vi "GEvt-Filter Global Log - v1.0.vi"(7 "Rules-v1":T1, 11 "Cross CSM Data (in)":T4) -> (0 "Matched? (dup)":bool, 3 "Cross CSM Data":T4)   [LabVIEW 2020, in "Communicable State Machine.lvlib"]
uses:
  Communicable State Machine.lvlib
  _CSM_GlobalLog_MSG.ctl
  _CSM_Response Source Message.ctl
  _CSM_GlobalLog_MSG_TYPE.ctl
  _CSM_GlobalLog Filter Rules - v1.0.ctl
  _CSM_GlobalLog_STATE_TYPE.ctl
  Set Global CSM Filter.vi
  Set Global LogType Filter.vi
  Set Global State Filter.vi
  Set CSM LogType Filter.vi
  Set CSM State Filter.vi
  Set Global StateType Filter.vi
  Set CSM StateType Filter.vi
  Group Check - CSM.vi
  Group Check - LogType.vi
  Group Check - State.vi
  CSM Check - LogType.vi
  CSM Check - State.vi
  CSM Check - StateType.vi
  Group Check - StateType.vi
  LogFilter.lvclass
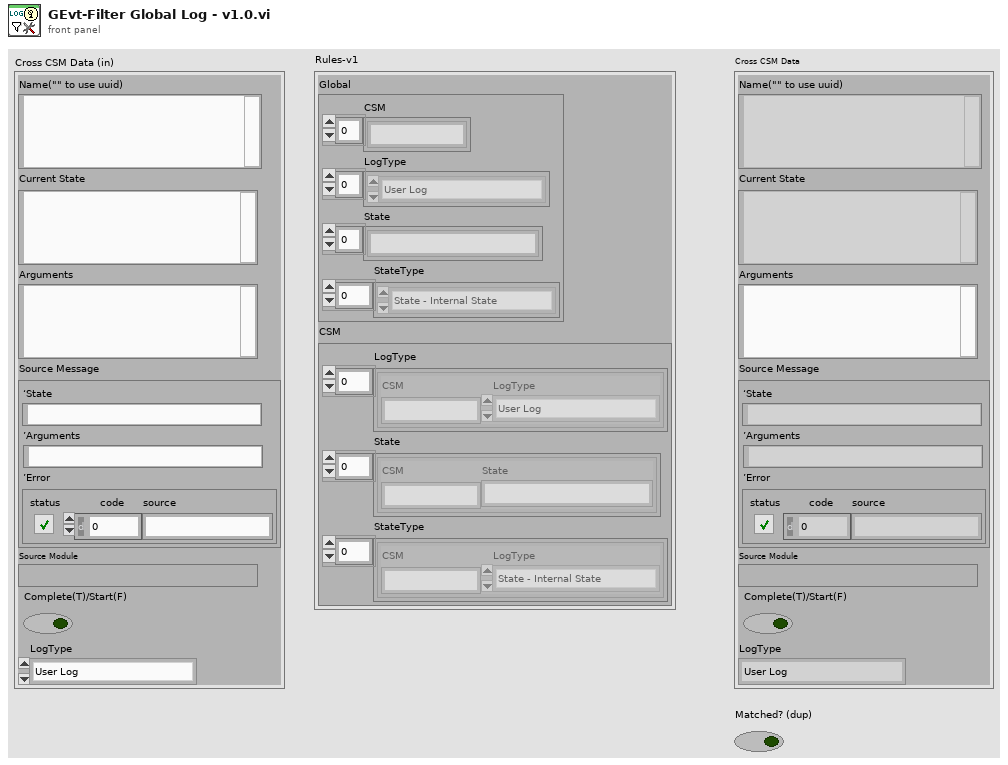
[diagram p1: front panel]
types:
  T1 = typedef "Communicable State Machine.lvlib/_CSM_GlobalLog Filter Rules - v1.0.ctl" = cluster{"Global":cluster{"CSM":string[], "LogType":T2[], "State":string[], "StateType":T3[]}, "CSM":cluster{"LogType":cluster{"CSM":string, "LogType":T2}[], "State":cluster{"CSM":string, "State":string}[], "StateType":cluster{"CSM":string, "LogType":T3}[]}}
  T2 = typedef "Communicable State Machine.lvlib/_CSM_GlobalLog_MSG_TYPE.ctl" = enum16{"User Log", "State Change", "Status", "Interrupt", "Register", "Unregister", "Error Log", "Module Created", "Module Destroyed"}
  T3 = typedef "Communicable State Machine.lvlib/_CSM_GlobalLog_STATE_TYPE.ctl" = enum16{"State - Internal State", "State - External Message", "State - Response", "State - Complete"}
  T4 = typedef "Communicable State Machine.lvlib/_CSM_GlobalLog_MSG.ctl" = cluster{"Name(\"\" to use uuid)":string, "Current State":string, "Arguments":string, "Source Message":T5, "Source Module":string, "Complete(T)/Start(F)":bool, "LogType":T2}
  T5 = typedef "Communicable State Machine.lvlib/_CSM_Response Source Message.ctl" = cluster{"‘State":string, "’Arguments":string, "’Error":errorcluster}
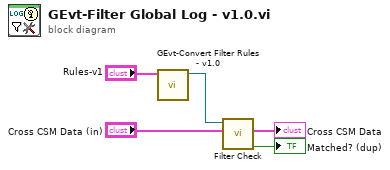
[diagram p0: block diagram]
diagram:
  n1 = call "GEvt-Convert Filter Rules - v1.0.vi"("Rules-v1"="Rules-v1") -> ("GlobalLogFilter"=w4:refnum<class "LogFilter.lvclass">)  [unwired: 10 in]
  n2 = call "Filter Check.vi"("Cross CSM Data in"="Cross CSM Data (in)", "GlobalLogFilter in"=w4) -> ("Matched? (dup)"=→"Matched? (dup)":bool, "Cross CSM Data out"=→"Cross CSM Data":T4)  [unwired: 7 in, 1 out]
